vi "View Data.vi"(1 "error in (no error)":errorcluster, 2 "Historic Data Input":T1) -> (0 "error out":errorcluster)   [LabVIEW 2021]
doc: "Visualiza los datos de temperatura adquiridos de una DAQ"
panel:
  in  "?":bool
  out "Historic Data":T1
  out "Temperature Data":T2(graph)
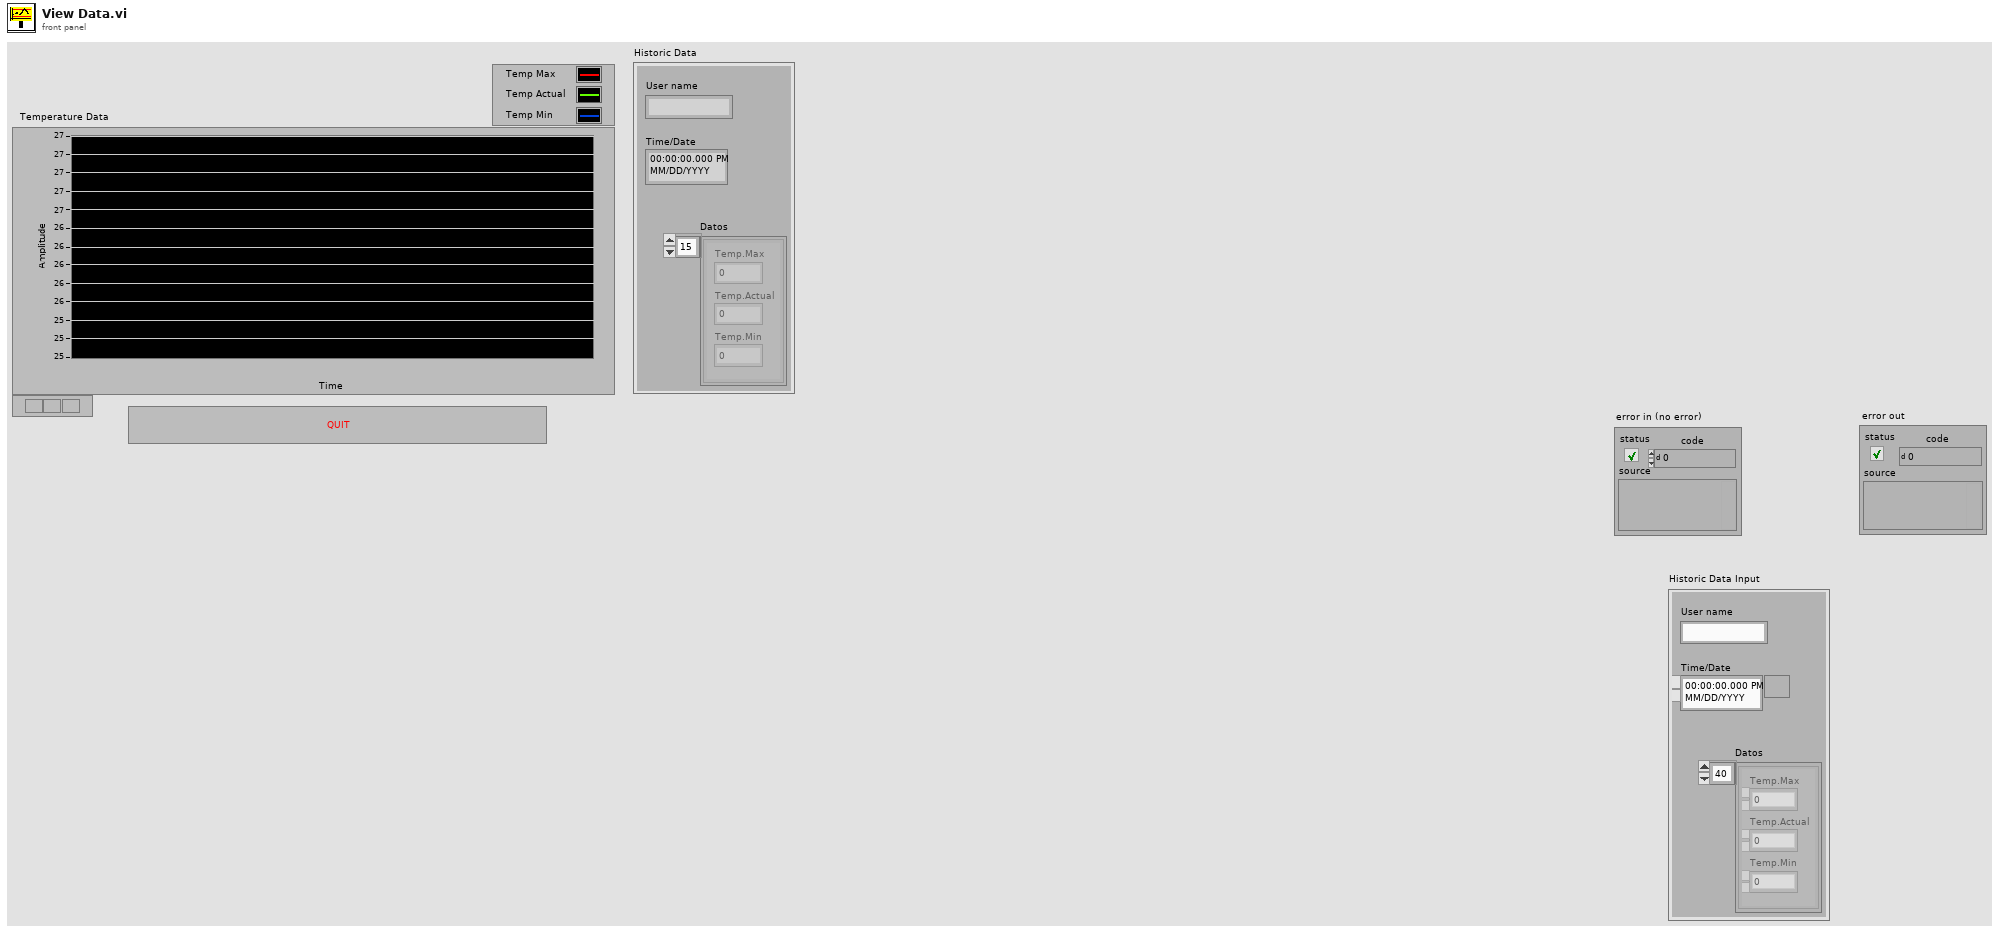
[diagram p1: front panel]
types:
  T1 = cluster{"User name":string, "Time/Date":timestamp, "Datos":cluster{"Temp.Max":dbl, "Temp.Actual":dbl, "Temp.Min":dbl}[]}
  T2 = cluster{"Temp.Max":dbl, "Temp.Actual":dbl, "Temp.Min":dbl}[]
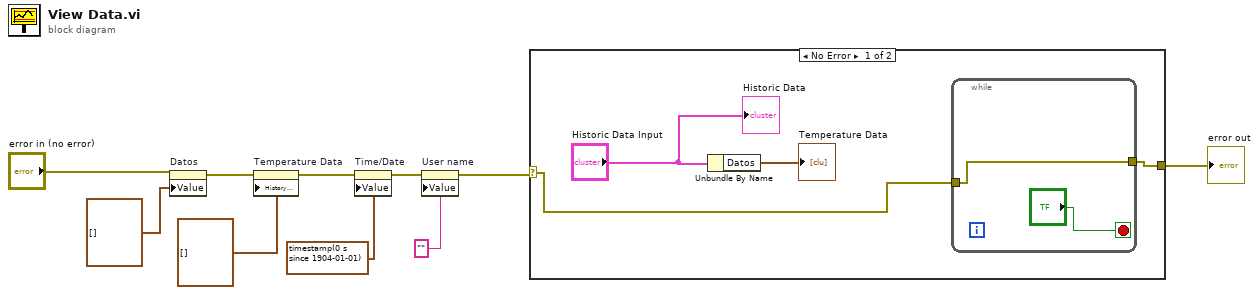
[diagram p0: block diagram]
diagram:
  n1 = property on="Datos" class="Arr (strict)"(error in="error in (no error)", "Value"=T2 []) -> (error out=w9:errorcluster)  [unwired: 1 in, 1 out]
  n2 = property on="Temperature Data" class="WFChart (strict)"(error in=w9, "History Data"=T2 []) -> (error out=w8:errorcluster)  [unwired: 1 in, 1 out]
  n3 = property on="Time/Date" class="AbsTime (strict)"(error in=w8, "Value"=timestamp(0 s since 1904-01-01)) -> (error out=w7:errorcluster)  [unwired: 1 in, 1 out]
  n4 = property on="User name" class="Str"(error in=w7, "Value"="") -> (error out=w2:errorcluster)  [unwired: 1 in, 1 out]
  n5 = case shown="No Error" w2 {
    selector: w2 -> [w12 w17]
    tunnel: [w11 w17] -> w1
    frame No Error {
      n6 = Unbundle By Name("Historic Data Input") -> ("Datos"=→"Temperature Data":T2)
      n7 = while {
        tunnel: w12 -> [w15]
        tunnel: [w15] -> w11
        stop <- "?" stop-if-true
      }
      "Historic Data" <- "Historic Data Input"
    }
    frame Error {
    }
  }
  "error out" <- w1
